vi "MoAgSy_GPG_deleteGpgFiles.vi"(0 "MoAgSy_GPG":refnum<class "MoAgSy_GPG.lvclass">, 1 "options file":path, 2 "keyringfile":path, 3 "Sec keyringfile":path, 5 "error in (no error)":errorcluster, 6 "Trust DB":path) -> (14 "dup MoAgSy_GPG":refnum<class "MoAgSy_GPG.lvclass">, 19 "error out":errorcluster)   [LabVIEW 2009, in "MoAgSy.lvlib" / "MoAgSy_GPG.lvclass"]
uses:
  MoAgSy_GPG.lvclass
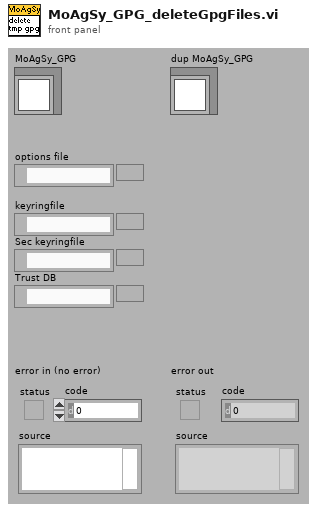
[diagram p1: front panel]
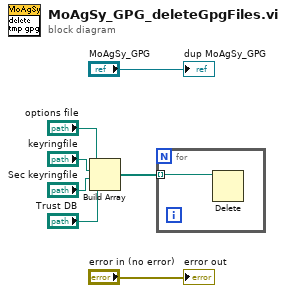
[diagram p0: block diagram]
diagram:
  n1 = Build Array("options file", "keyringfile", "Sec keyringfile", "Trust DB") -> (w1:path[])
  n2 = for {
    tunnel: w1 -> [w8] mode=indexing
    n3 = Delete(path (use dialog)=w8) -> ()  [unwired: 1 in, 6 out]
  }
  "error out" <- "error in (no error)"
  "dup MoAgSy_GPG" <- "MoAgSy_GPG"
